vi "Ustawienie położenia z uwzględnieniem położenia początkowego i przesunięcia.vi"(10 "Poł. startowe":cluster{"Piksel x":i32, "Piksel y":i32}, 11 "Przesunięcie mapy":cluster{"X":i16, "Y":i16}) -> (3 "Początkowe położenie robota out":cluster{"X":i16, "Y":i16})   [LabVIEW 2012, in "Biblioteka moduł map v3.lvlib" / "Obsługa grafiki mapy.lvlib"]
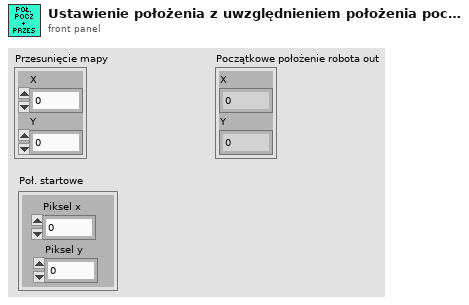
[diagram p1: front panel]
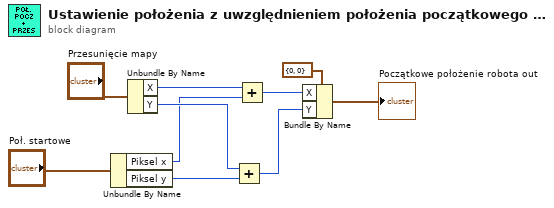
[diagram p0: block diagram]
diagram:
  n1 = Unbundle By Name("Poł. startowe") -> ("Piksel x"=w2:i32, "Piksel y"=w1:i32)
  n2 = Unbundle By Name("Przesunięcie mapy") -> ("X"=w7:i16, "Y"=w10:i16)
  n3 = Add(x=w10, y=w1) -> (x+y=w9:i32)
  n4 = Add(x=w7, y=w2) -> (x+y=w8:i32)
  n5 = Bundle By Name(cluster=cluster{"X":i16, "Y":i16} {"X"=0, "Y"=0} ("Początkowe położenie robota"), "X"=w8, "Y"=w9) -> (→"Początkowe położenie robota out":cluster{"X":i16, "Y":i16})
